vi "Example.vi"() -> ()   [LabVIEW 2015, in "RealTimeFilter.lvlib"]
uses:
  TypeDefs/Modes.ctl
  <vilib>/Platform/TimedLoop/XDataNode/timing_clust.ctl
  <vilib>/Platform/TimedLoop/XDataNode/nitl_modes.ctl
  <vilib>/Platform/TimedLoop/XDataNode/wakeup.ctl
  <vilib>/platform/TimedLoop/XDataNode/XDataNode.xnode
  RealTimeFilter.lvlib
  <vilib>/Platform/TimedLoop/XDataNode/XDNodeRunTimeDep.lvlib
panel:
  out "Jerk":cluster{"filtered signal":dbl, "demand":dbl}(graph)
  out "Acceleration":cluster{"filtered signal":dbl, "demand":dbl}(graph)
  in  "demand":dbl(slide)=1.0 scale=0.0..10.0
  out "Speed":cluster{"filtered signal":dbl, "demand":dbl}(graph)
  in  "stop":bool
  in  "gaussian stdev":dbl=7.0
  in  "number of elements":i32=50
  out "Input vs output":cluster{"filtered signal":dbl, "demand":dbl}(graph)
  in  "max speed":dbl(slide)=1.0 scale=0.0..0.1
  in  "Mode":T1
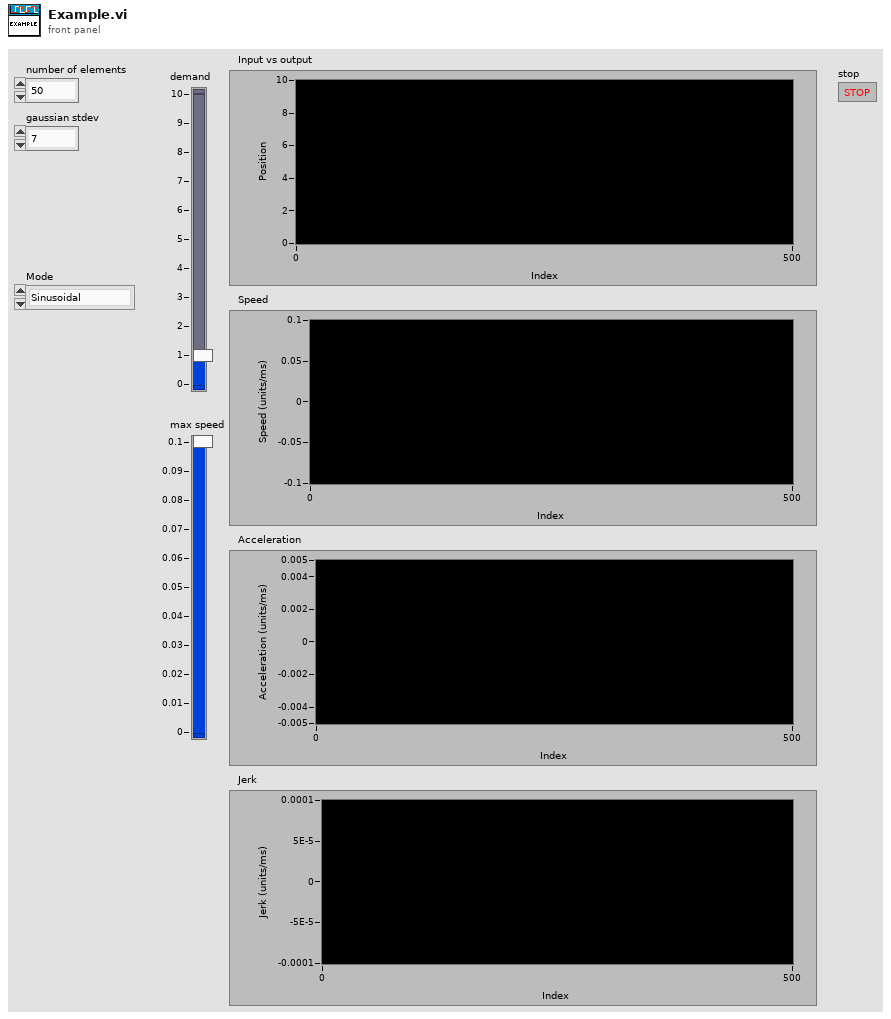
[diagram p1: front panel]
types:
  T1 = typedef "RealTimeFilter.lvlib/Modes.ctl" = enum16{"Sinusoidal", "Gaussian"}
  T2 = typedef "RealTimeFilter.lvlib/Parameters.ctl" = cluster{"number of elements":i32, "start value":dbl, "sinusoidal profile":dbl[], "gaussian profile":dbl[]}
  T3 = typedef "XDNodeRunTimeDep.lvlib/timing_clust.ctl" = cluster{"Expected End [f-1]":u64, "Actual End [f-1]":u64, "Finished Late? [f-1]":bool, "Expected End [i-1]":u64, "Actual End [i-1]":u64, "Finished Late? [i-1]":bool, "Expected Start [i]":u64, "Actual Start [i]":u64, "Expected Start [f]":u64, "Actual Start [f]":u64, "Source Name":string, "Structure Name":string, "Period":i64, "Deadline":i64, "Offset":i64, "Start":i64, "Priority":i32, "Timeout":i32, "Mode":T4, "Wakeup Reason":T5, "Error":errorcluster, "Source Type":string, "Secondary Source Type":string, "Global End Time":u64, "Global Start Time":u64, "Frame Duration":u64, "Iteration Duration":u64, "Assigned CPU":i32, "I/O Scan Engine Mode":u32}
  T4 = typedef "XDNodeRunTimeDep.lvlib/nitl_modes.ctl" = enum32{"No Change", "Process missed periods, maintain original phase", "Discard missed periods, maintain original phase", "Process missed periods, ignore original phase", "Discard missed periods, ignore original phase"}
  T5 = typedef "XDNodeRunTimeDep.lvlib/wakeup.ctl" = enum32{"Normal", "Aborted", "Asynchronous wakeup", "Timing source error", "Timed loop error", "Timeout"}
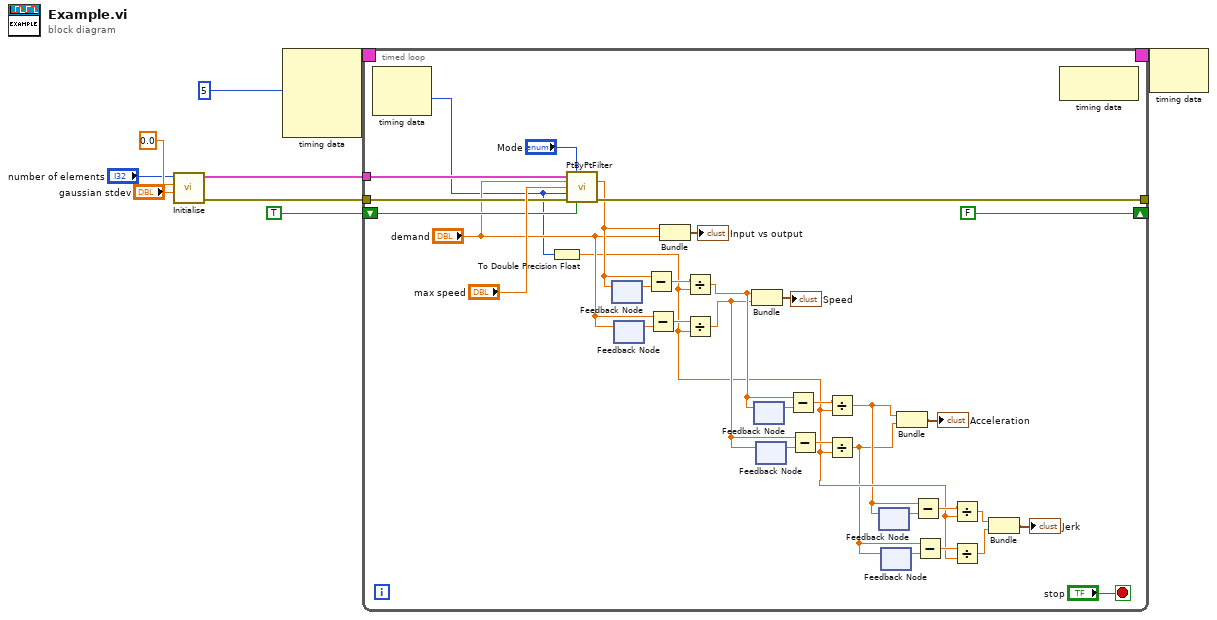
[diagram p0: block diagram]
diagram:
  n1 = call "Initialise.vi"("gaussian stdev (elements)"="gaussian stdev", "start value"=0.0, "number of elements (max 2048)"="number of elements") -> ("error out"=w5:errorcluster, "parameter cluster"=w6:T2)  [unwired: 7 in]
  n2 = node-c288(i64 5 ("Period")) -> (w9:T3)  [unwired: 3 in]
  n3 = timed-loop {
    timing: w9 -> [_]
    timing-out: [_] -> w8
    tunnel: w6 -> [w43]
    tunnel: w5 -> [w40]
    tunnel: [w39] -> _
    shift-right: [FALSE ("stop")] -> _
    shift-left: TRUE ("stop") -> [w35]
    stop <- "stop" stop-if-true
    n4 = node-c288() -> (w20:i64)  [unwired: 1 in, 1 out]
    n5 = To Double Precision Float(number=w20) -> (double precision float=w12:dbl)
    n6 = call "PtByPtFilter.vi"("parameter cluster"=w43, "Mode"="Mode", "demand"="demand", "max speed"="max speed", "dt"=w20, "error in"=w40, "reset"=w35) -> ("filtered signal"=w33:dbl, "error out"=w39:errorcluster)  [unwired: 7 in]
    n7 = feedback-in #1(w33) -> ()
    n8 = feedback #1() -> (w34:dbl)  [unwired: 1 in]
    n9 = feedback #2() -> (w32:dbl)  [unwired: 1 in]
    n10 = feedback-in #2("demand") -> ()
    n11 = Subtract(x=w33, y=w34) -> (x-y=w29:dbl)
    n12 = Subtract(x="demand", y=w32) -> (x-y=w28:dbl)
    n13 = Bundle("filtered signal"=w33, "demand"="demand") -> (→"Input vs output":cluster{"filtered signal":dbl, "demand":dbl})  [unwired: 1 in]
    n14 = Divide(x=w29, y=w12) -> (x/y=w22:dbl)
    n15 = Divide(x=w28, y=w12) -> (x/y=w21:dbl)
    n16 = Bundle(w22, w21) -> (→"Speed":cluster{dbl, dbl})  [unwired: 1 in]
    n17 = feedback #3() -> (w23:dbl)  [unwired: 1 in]
    n18 = feedback-in #3(w22) -> ()
    n19 = feedback #4() -> (w24:dbl)  [unwired: 1 in]
    n20 = feedback-in #4(w21) -> ()
    n21 = Subtract(x=w22, y=w23) -> (x-y=w26:dbl)
    n22 = Subtract(x=w21, y=w24) -> (x-y=w27:dbl)
    n23 = Divide(x=w26, y=w12) -> (x/y=w11:dbl)
    n24 = Divide(x=w27, y=w12) -> (x/y=w10:dbl)
    n25 = feedback #5() -> (w19:dbl)  [unwired: 1 in]
    n26 = feedback-in #5(w11) -> ()
    n27 = feedback #6() -> (w18:dbl)  [unwired: 1 in]
    n28 = feedback-in #6(w10) -> ()
    n29 = Bundle(w11, w10) -> (→"Acceleration":cluster{dbl, dbl})  [unwired: 1 in]
    n30 = Subtract(x=w11, y=w19) -> (x-y=w16:dbl)
    n31 = Subtract(x=w10, y=w18) -> (x-y=w15:dbl)
    n32 = Divide(x=w16, y=w12) -> (x/y=w14:dbl)
    n33 = Divide(x=w15, y=w12) -> (x/y=w13:dbl)
    n34 = Bundle(w14, w13) -> (→"Jerk":cluster{dbl, dbl})  [unwired: 1 in]
    n35 = node-c288() -> ()  [unwired: 1 in, 1 out]
  }
  n36 = node-c288(w8) -> ()  [unwired: 1 out]
